vi "ma_Force Restart (2ch) no State.vi"(0 "averaging parameters":T3={"averaging mode"=enum."No averaging", "weighting mode"=enum."Exponential", "number of averages"=10} {"number of averages" min=1}, 1 "force restart averaging in":bool, 5 "window":T2=1 items=["Rectangle"=0, "Hanning"=1, "Hamming"=2, "Blackman-Harris"=3, "Exact Blackman"=4, "Blackman"=5, "Flat Top"=6, "4 Term B-Harris "=7, "7 Term B-Harris"=8, "Low Sidelobe"=9, "Blackman Nuttall"=11, "Triangle"=30, "Bartlett-Hanning"=31, "Bohman"=32, "Parzen"=33, "Welch"=34, "Kaiser"=60, "Dolph-Chebyshev"=61, "Gaussian"=62], 9 "restart averaging (F)":bool, 12 "caller VI name":string, 13 "state info":T1 {"Syy" format="%0.2f"; "Sxy" format="%0.2f"; "Sy" format="%0.2f"; "Sxx" format="%0.2f"; "avgs completed" format="%0.2f"; "df" format="%0.2f"; "Sx" format="%0.2f"; "spectrum parameters"."window" items=["Rectangle"=0, "Hanning"=1, "Hamming"=2, "Blackman-Harris"=3, "Exact Blackman"=4, "Blackman"=5, "Flat Top"=6, "4 Term B-Harris "=7, "7 Term B-Harris"=8, "Low Sidelobe"=9, "Blackman Nuttall"=11, "Triangle"=30, "Bartlett-Hanning"=31, "Bohman"=32, "Parzen"=33, "Welch"=34, "Kaiser"=60, "Dolph-Chebyshev"=61, "Gaussian"=62]; "dt" format="%0.2f"; "timestamp" format="%0.2f"; "dt history" format="%0.2f"; "t0 history" format="%0.2f"}) -> (4 "skip processing":errorcluster, 6 "force restart averaging":bool, 10 "retrieve last spectrum":bool, 14 "state info out":T1 {"Syy" format="%0.2f"; "Sxy" format="%0.2f"; "Sy" format="%0.2f"; "Sxx" format="%0.2f"; "avgs completed" format="%0.2f"; "df" format="%0.2f"; "Sx" format="%0.2f"; "spectrum parameters"."window" items=["Rectangle"=0, "Hanning"=1, "Hamming"=2, "Blackman-Harris"=3, "Exact Blackman"=4, "Blackman"=5, "Flat Top"=6, "4 Term B-Harris "=7, "7 Term B-Harris"=8, "Low Sidelobe"=9, "Blackman Nuttall"=11, "Triangle"=30, "Bartlett-Hanning"=31, "Bohman"=32, "Parzen"=33, "Welch"=34, "Kaiser"=60, "Dolph-Chebyshev"=61, "Gaussian"=62]; "dt" format="%0.2f"; "timestamp" format="%0.2f"; "dt history" format="%0.2f"; "t0 history" format="%0.2f"}, 15 "error out":errorcluster)   [LabVIEW 2020, in "NI_MAPro.lvlib"]
uses:
  NI_MAPro.lvlib
  windowTd.ctl
  2-chan State.ctl
  NI_AALPro.lvlib
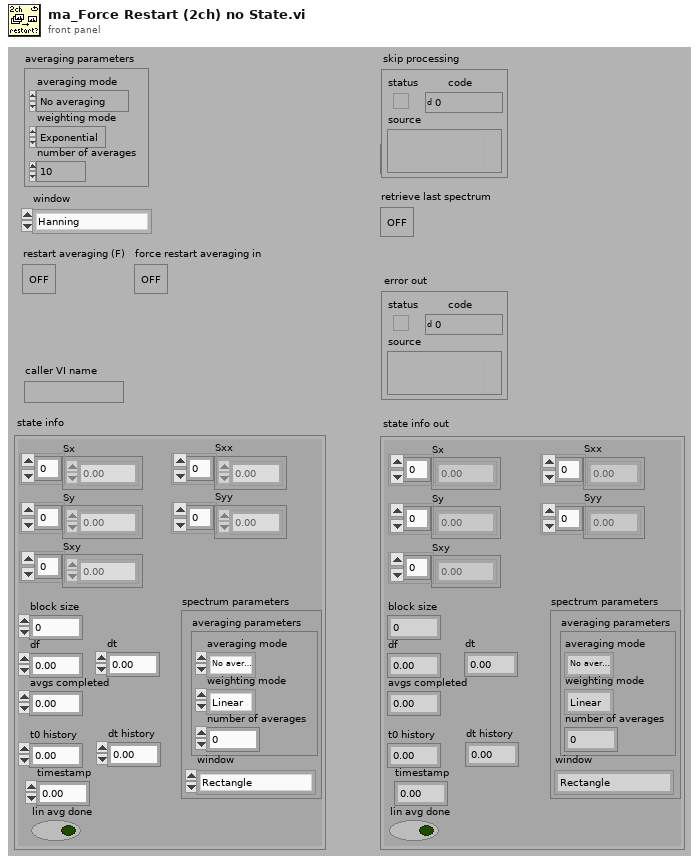
[diagram p1: front panel]
types:
  T1 = typedef "NI_MAPro.lvlib/2-chan State.ctl" = cluster{"Sx":cdb[], "Sy":cdb[], "Sxx":dbl[], "Syy":dbl[], "Sxy":cdb[], "block size":i32, "df":dbl, "dt":dbl, "avgs completed":dbl, "spectrum parameters":cluster{"averaging parameters":cluster{"averaging mode":enum16{"No averaging", "Vector averaging", "RMS averaging", "Peak hold"}, "weighting mode":enum16{"Linear", "Exponential"}, "number of averages":u32}, "window":T2}, "lin avg done":bool, "t0 history":dbl, "dt history":dbl, "timestamp":dbl}
  T2 = typedef "NI_AALPro.lvlib/windowTd.ctl" = u32
  T3 = cluster{"averaging mode":enum16{"No averaging", "Vector averaging", "RMS averaging", "Peak hold"}, "weighting mode":enum16{"Linear", "Exponential"}, "number of averages":u32}
  T4 = cluster{"averaging parameters":cluster{"averaging mode":enum16{"No averaging", "Vector averaging", "RMS averaging", "Peak hold"}, "weighting mode":enum16{"Linear", "Exponential"}, "number of averages":u32}, "window":T2}
  T5 = enum16{"No averaging", "Vector averaging", "RMS averaging", "Peak hold"}
  T6 = cluster{"status":bool, "code":i32, "caller VI name":string}
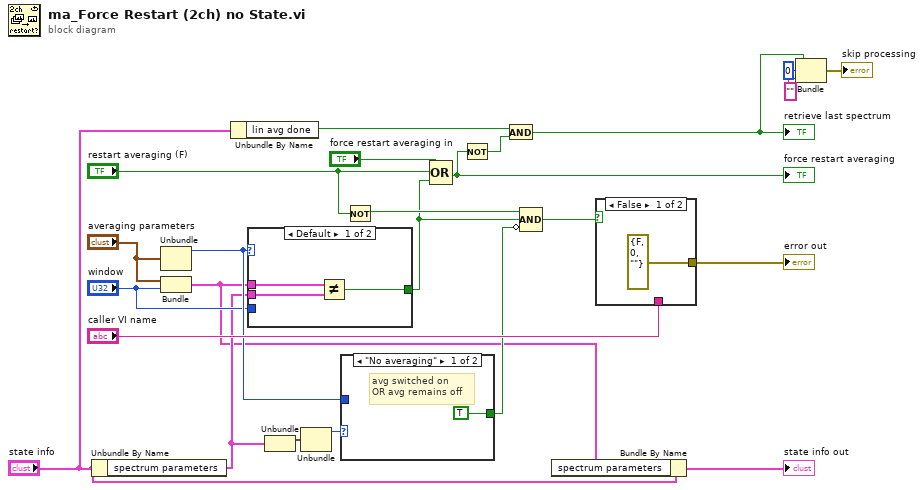
[diagram p0: block diagram]
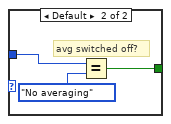
[diagram p2: hidden frame]
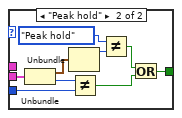
[diagram p3: hidden frame]
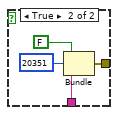
[diagram p4: hidden frame]
diagram:
  n1 = Unbundle By Name("state info") -> ("spectrum parameters"=w5:T4)
  n2 = Unbundle("averaging parameters") -> ("averaging mode"=w16:T5)  [unwired: 2 out]
  n3 = Bundle("averaging parameters"="averaging parameters", "window"="window") -> (w4:T4)  [unwired: 1 out]
  n4 = Unbundle By Name("state info") -> ("lin avg done"=w1:bool)
  n5 = case shown="Default" w16 {
    tunnel: w5 -> [w27 w36]
    tunnel: [w26 w30] -> w10
    tunnel: w4 -> [w25 _]
    tunnel: "window" -> [_ w34]
    frame Default {
      n6 = Not Equal?(x=w25, y=w27) -> (x != y?=w26:bool)
    }
    frame "Peak hold" {
      n7 = Unbundle(w36) -> ("averaging parameters"=w33:T3, "window"=w35:T2)
      n8 = Unbundle(w33) -> ("averaging mode"=w29:T5)  [unwired: 2 out]
      n9 = Not Equal?(x=w35, y=w34) -> (x != y?=w31:bool)
      n10 = Not Equal?(x=T5."Peak hold" ("y"), y=w29) -> (x != y?=w32:bool)
      n11 = Or(x=w32, y=w31) -> (x .or. y?=w30:bool)
    }
  }
  n12 = Unbundle(w5) -> ("averaging parameters"=w8:T3)  [unwired: 1 out]
  n13 = Unbundle(w8) -> ("averaging mode"=w6:T5)  [unwired: 2 out]
  n14 = case shown="\"No averaging\"" w6 {
    tunnel: w16 -> [_ w40]
    tunnel: [TRUE w38] -> w7
    frame "No averaging" {
      # "avg switched on \nOR avg remains off"
    }
    frame Default {
      # "avg switched off?"
      n15 = Equal?(x=w40, y=T5."No averaging" ("averaging mode")) -> (x = y?=w38:bool)
    }
  }
  n16 = Not(x="restart averaging (F)") -> (.not. x?=w11:bool)
  n17 = Compound Arithmetic op=OR("force restart averaging in", "restart averaging (F)", w10) -> (w23:bool)
  "force restart averaging" <- w23
  n18 = Not(x=w23) -> (.not. x?=w13:bool)
  n19 = And(x=w1, y=w13) -> (x .and. y?=w19:bool)
  "retrieve last spectrum" <- w19
  n20 = Compound Arithmetic op=AND(w11, w10, invert w7) -> (w9:bool)
  n21 = Bundle By Name(cluster="state info", "spectrum parameters"=w4) -> (→"state info out":T1)
  n22 = case shown="False" w9 {
    tunnel: [errorcluster {"status"=FALSE, "code"=0, "source"=""} ("error out") w45] -> w18
    tunnel: "caller VI name" -> [_ w42]
    frame False {
    }
    frame True {
      n23 = Bundle("status"=FALSE, "code"=20351, "caller VI name"=w42) -> (w45:T6)  [unwired: 1 out]
    }
  }
  "error out" <- w18
  n24 = Bundle(w19, "code"=0, "source"="") -> (→"skip processing":cluster{bool, "code":i32, "source":string})  [unwired: 1 out]
